vi "Update_Results_file_copies.vi"(2 "Raw data option":enum16{"Save raw data", "Raw data not saved"}(ring), 4 "Raw data file":path, 5 "Results file":path) -> ()   [LabVIEW 2010]
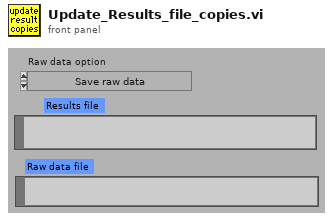
[diagram p1: front panel]
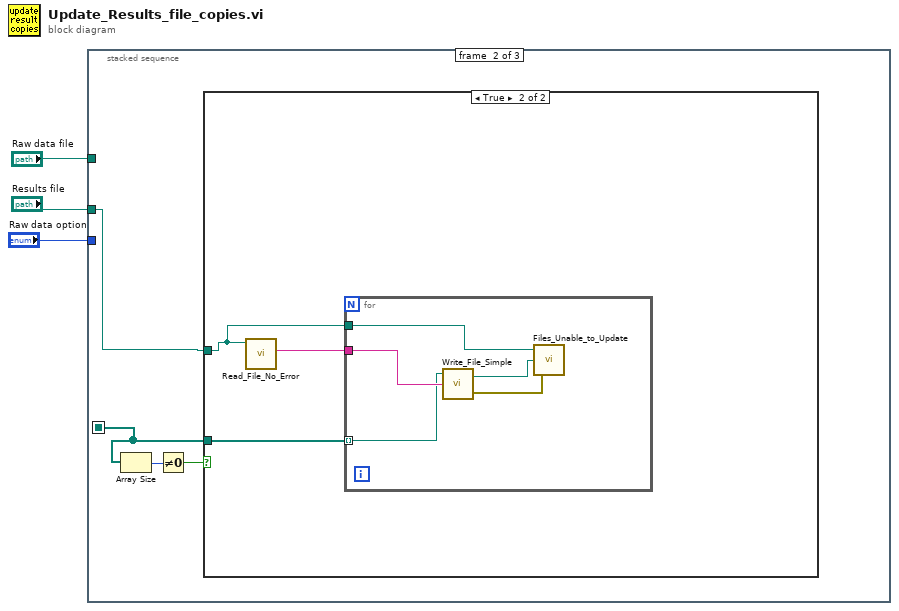
[diagram p0: block diagram]
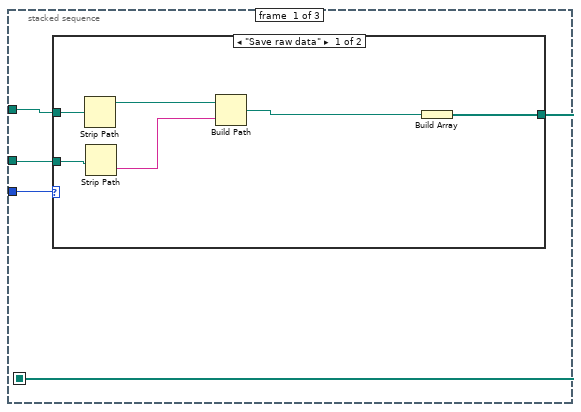
[diagram p2: hidden frame]
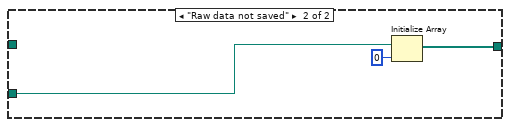
[diagram p3: hidden frame]
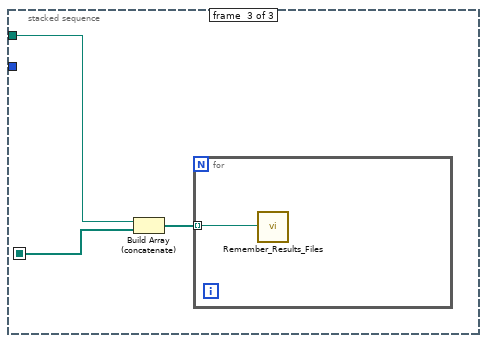
[diagram p5: hidden frame]
diagram:
  n1 = stacked-sequence {
    seq-local: [w4 _ _] -> [_ w17 w29]
    tunnel: "Results file" -> [w7 w18 w30]
    tunnel: "Raw data file" -> [w6 _ _]
    tunnel: "Raw data option" -> [w5 _ _]
    frame #0 {
      n2 = case shown="\"Save raw data\"" w5 {
        tunnel: w6 -> [w11 _]
        tunnel: w7 -> [w12 w14]
        tunnel: [w13 w15] -> w4
        frame "Save raw data" {
          n3 = Strip Path(path=w11) -> (stripped path=w10:path)  [unwired: 1 out]
          n4 = Strip Path(path=w12) -> (name=w9:string)  [unwired: 1 out]
          n5 = Build Path(base path=w10, name or relative path=w9) -> (appended path=w8:path)
          n6 = Build Array(w8) -> (w13:path[])
        }
        frame "Raw data not saved" {
          n7 = Initialize Array(w14, 0 ("Dimension Size")) -> (w15:path[])
        }
      }
    }
    frame #1 {
      n8 = Array Size(array=w17) -> (size(s)=w20:i32)
      n9 = Not Equal To 0?(x=w20) -> (x != 0?=w19:bool)
      n10 = case shown="True" w19 {
        tunnel: w18 -> [_ w21]
        tunnel: w17 -> [_ w23]
        frame False {
        }
        frame True {
          n11 = call "Read_File_No_Error.vi"("Filename"=w21) -> ("string"=w22:string)  [unwired: 2 in, 7 out]
          n12 = for {
            tunnel: w23 -> [w24] mode=indexing
            tunnel: w22 -> [w28]
            tunnel: w21 -> [w25]
            n13 = call "Write_File_Simple.vi"("character string"=w28, "file path"=w24) -> ("error out"=w26:errorcluster, "file path Out"=w27:path)  [unwired: 1 in]
            n14 = call "Files_Unable_to_Update.vi"("error in (no error)"=w26, "Target Path"=w27, "Source Path"=w25) -> ()  [unwired: 1 out]
          }
        }
      }
    }
    frame #2 {
      n15 = Build Array (concatenate)(w30, w29) -> (w31:path[])
      n16 = for {
        tunnel: w31 -> [w32] mode=indexing
        n17 = call "Remember_Results_Files.vi"("Filename to Remember"=w32) -> ()  [unwired: 1 out]
      }
    }
  }
